vi "Untitled 2 (SubVI).vi"(0 "ROI Descriptor COLOR Mask":T1={"Global Rectangle"=[109, 72, 345, 284], "Contours"=[{"ID"=enum."External", "Type"=3, "Coordinates"=[109, 72, 345, 284]}]} {"Contours"."Type" items=["No Selection", "Point", "Line", "Rectangle", "Oval", "Polygon", "Freehand Region", "Annulus", "Unused2", "Unused3", "Broken Line", "Freehand Line", "Rotated Rectangle"]}, 1 "reference 3":refnum<vi>, 2 "reference in":refnum<vi>, 7 "Ball index":i32, 9 "Boolean":bool, 12 "CircleRadius":dbl, 13 "divider (circle)":sgl) -> (4 "ROI Descriptor COLOR Mask out":T1={"Global Rectangle"=[109, 72, 345, 284], "Contours"=[{"ID"=enum."External", "Type"=3, "Coordinates"=[109, 72, 345, 284]}]} {"Contours"."Type" items=["No Selection", "Point", "Line", "Rectangle", "Oval", "Polygon", "Freehand Region", "Annulus", "Unused2", "Unused3", "Broken Line", "Freehand Line", "Rotated Rectangle"]}, 6 "index 2":i32, 8 "index":i32, 10 "index 3":i32, 14 "index 4":i32)   [LabVIEW 2017]
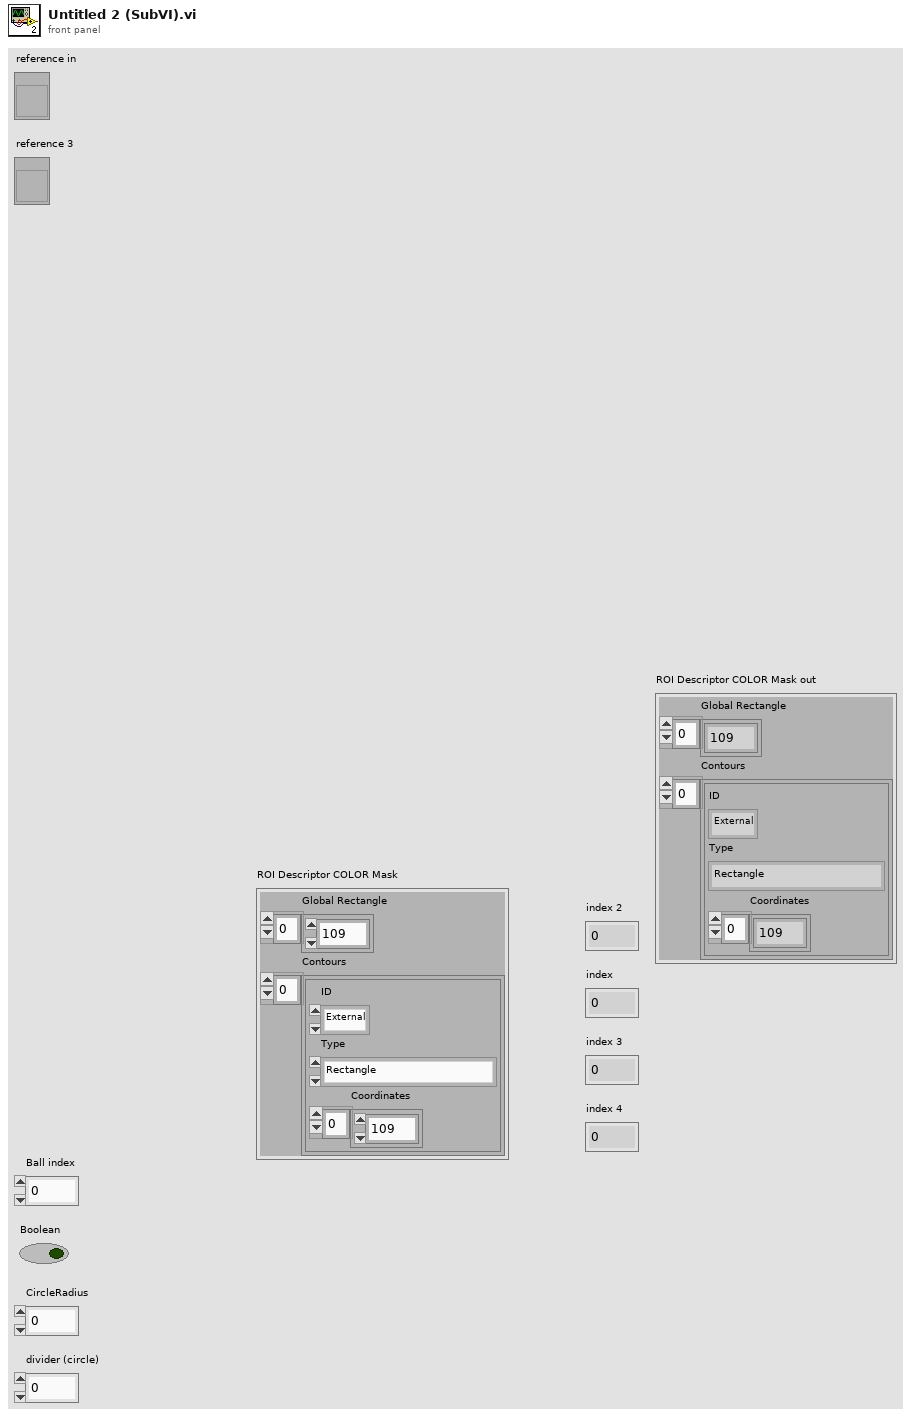
[diagram p1: front panel]
types:
  T1 = cluster{"Global Rectangle":i32[], "Contours":cluster{"ID":enum32{"External", "Internal"}, "Type":u32, "Coordinates":i32[]}[]}
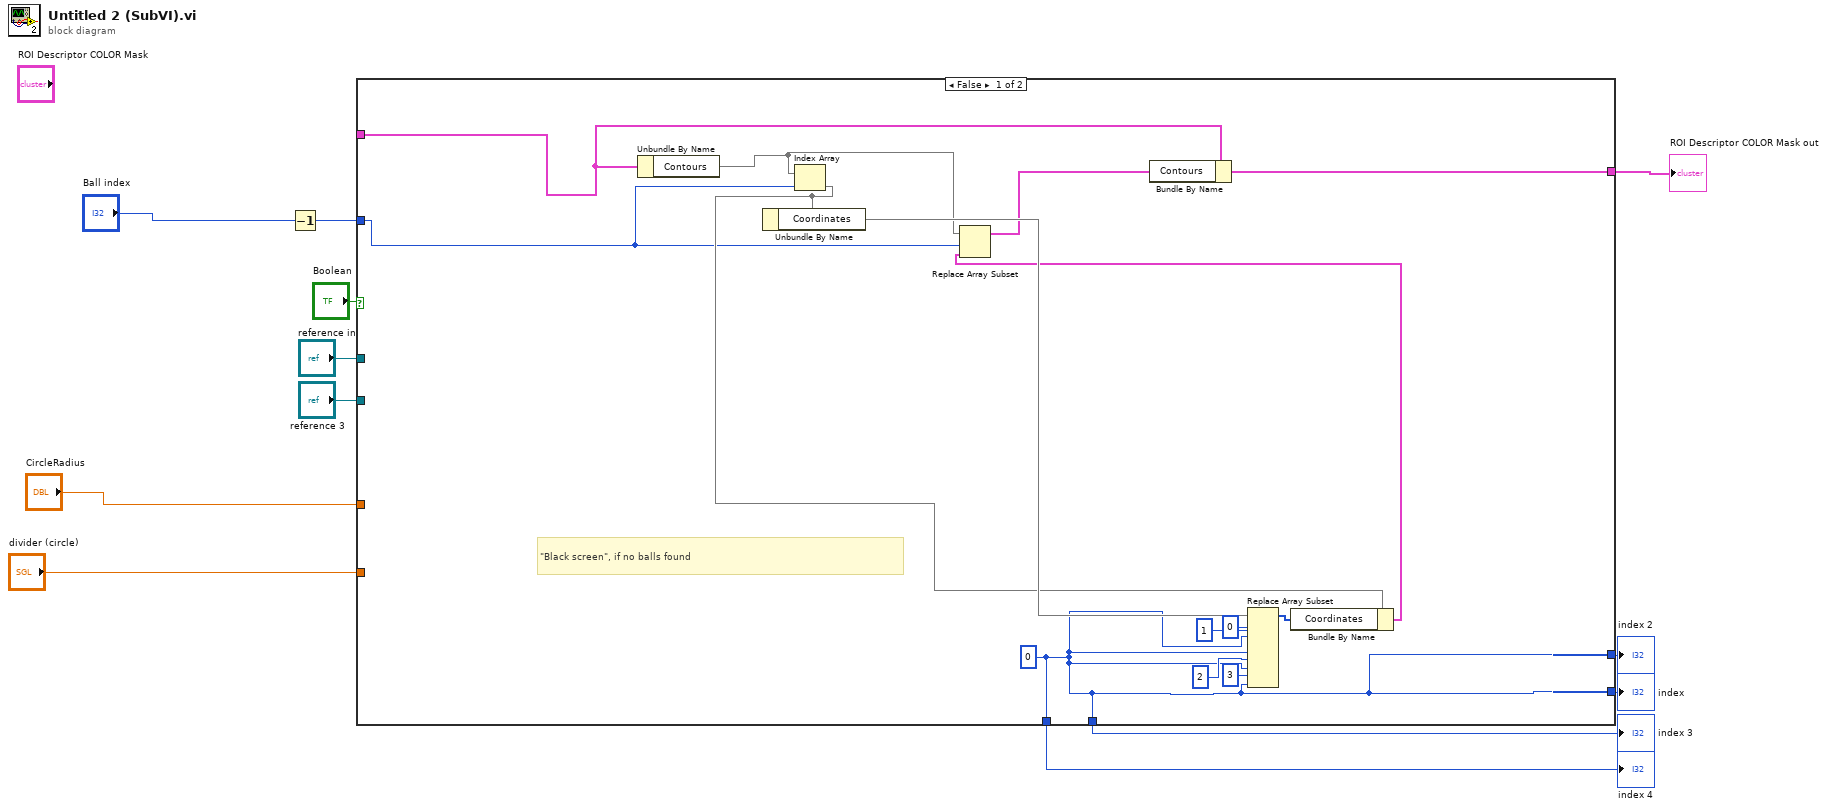
[diagram p0: block diagram]
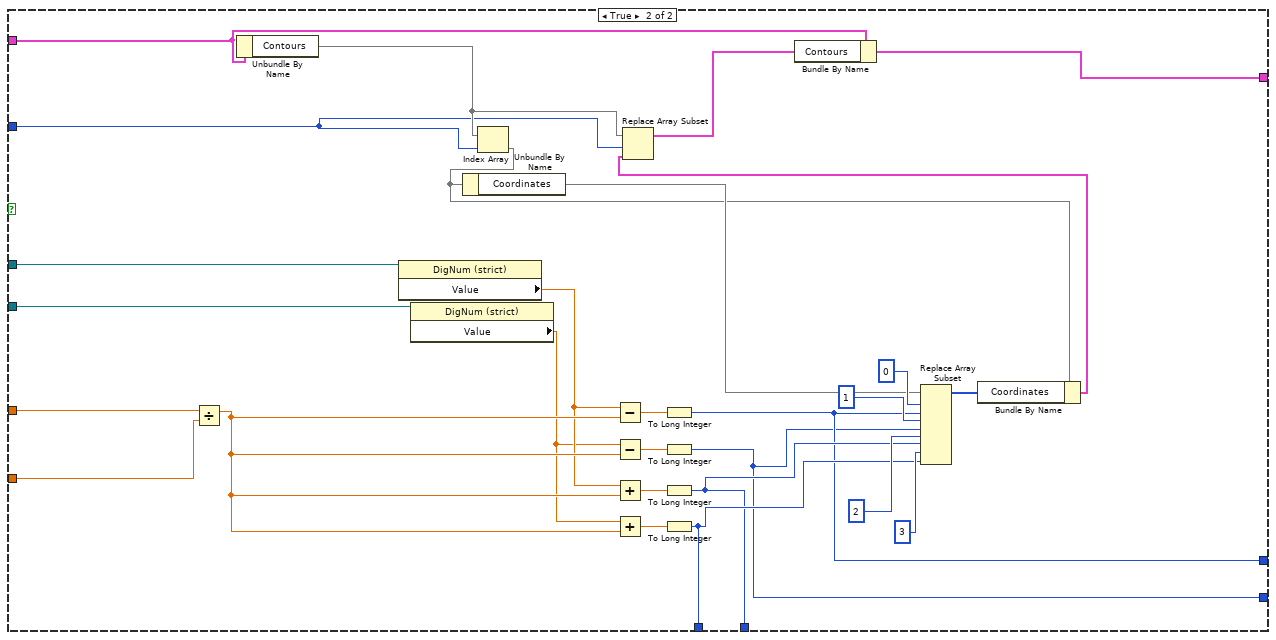
[diagram p2: hidden frame]
diagram:
  n1 = Decrement(x="Ball index") -> (x-1=w1:i32)
  n2 = case shown="False" "Boolean" {
    tunnel: "divider (circle)" -> [_ w38]
    tunnel: w1 -> [w16 w37]
    tunnel: [w17 w36] -> w9
    tunnel: [w17 w35] -> w10
    tunnel: [w17 w34] -> w11
    tunnel: [w17 w33] -> w12
    tunnel: "CircleRadius" -> [_ w32]
    tunnel: "reference in" -> [_ w31]
    tunnel: "reference 3" -> [_ w30]
    tunnel: _ -> [w15 w28]
    tunnel: [w14 w29] -> w2
    frame False {
      w17 = 0 ("index")
      # "\"Black screen\", if no balls found"
      n3 = Unbundle By Name(w15) -> ("Contours"=w18)
      n4 = Index Array(array=w18, index=w16) -> (element=w22)
      n5 = Unbundle By Name(w22) -> ("Coordinates"=w23)
      n6 = Replace Array Subset(array=w23, new element #1=w17, index #1=0 ("index"), new element #2=w17, index #2=1 ("index"), new element #3=w17, index #3=2 ("index"), new element #4=w17, index #4=3 ("index")) -> (w20:i32[])
      n7 = Bundle By Name(cluster=w22, "Coordinates"=w20) -> (w21:cluster{})
      n8 = Replace Array Subset(array=w18, new element=w21, index=w16) -> (w19:cluster{}[])
      n9 = Bundle By Name(cluster=w15, "Contours"=w19) -> (w14:cluster{})
    }
    frame True {
      n10 = Divide(x=w32, y=w38) -> (x/y=w51:dbl)
      n11 = Unbundle By Name(w28) -> ("Contours"=w42)
      n12 = property class="DigNum (strict)"(reference=w31) -> ("Value"=w40:sgl)  [unwired: 1 in, 2 out]
      n13 = property class="DigNum (strict)"(reference=w30) -> ("Value"=w39:sgl)  [unwired: 1 in, 2 out]
      n14 = Index Array(array=w42, index=w37) -> (element=w45)
      n15 = Unbundle By Name(w45) -> ("Coordinates"=w46)
      n16 = Subtract(x=w40, y=w51) -> (x-y=w55:dbl)
      n17 = Subtract(x=w39, y=w51) -> (x-y=w54:dbl)
      n18 = Add(x=w40, y=w51) -> (x+y=w52:dbl)
      n19 = Add(x=w39, y=w51) -> (x+y=w53:dbl)
      n20 = To Long Integer(number=w55) -> (32bit integer=w34:i32)
      n21 = To Long Integer(number=w54) -> (32bit integer=w33:i32)
      n22 = To Long Integer(number=w52) -> (32bit integer=w35:i32)
      n23 = To Long Integer(number=w53) -> (32bit integer=w36:i32)
      n24 = Replace Array Subset(array=w46, new element #1=w34, index #1=0 ("index"), new element #2=w33, index #2=1 ("index"), new element #3=w35, index #3=2 ("index"), new element #4=w36, index #4=3 ("index")) -> (w43:i32[])
      n25 = Bundle By Name(cluster=w45, "Coordinates"=w43) -> (w44:cluster{})
      n26 = Replace Array Subset(array=w42, new element=w44, index=w37) -> (w41:cluster{}[])
      n27 = Bundle By Name(cluster=w28, "Contours"=w41) -> (w29:cluster{})
    }
  }
  "index" <- w12
  "index 2" <- w11
  "index 3" <- w10
  "index 4" <- w9
  "ROI Descriptor COLOR Mask out" <- w2
